vi "FGV Rel.vi"(5 "Extrem_Value":T1, 9 "action":enum16{"set", "get"}(ring), 11 "error in (no error)":errorcluster) -> (6 "Extrem_Value":T1, 15 "error out":errorcluster)   [LabVIEW 2014, in "FH 55.lvlib"]
uses:
  FH 55.lvlib
  TypeDef/Value_String.ctl
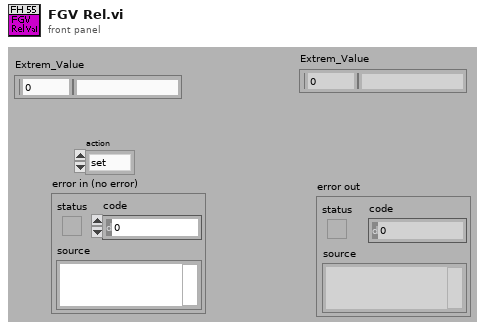
[diagram p1: front panel]
types:
  T1 = typedef "FH 55.lvlib/Value_String.ctl" = cluster{"Numeric":dbl, "String":string}
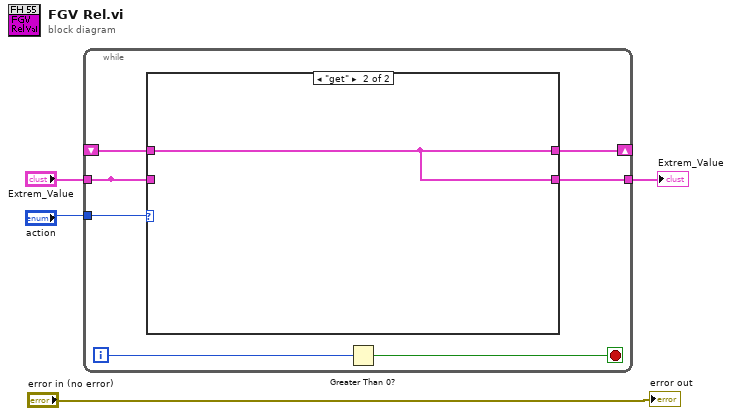
[diagram p0: block diagram]
diagram:
  n1 = while {
    tunnel: "Extrem_Value" -> [w10]
    tunnel: [w10] -> _
    shift-right: [w8] -> _
    shift-left: _ -> [w11]
    tunnel: [w9] -> w2
    tunnel: "action" -> [w5]
    i -> [w7]
    stop <- w6 stop-if-true
    n2 = case shown="\"get\"" w5 {
      tunnel: w11 -> [_ w13]
      tunnel: w10 -> [w12 _]
      tunnel: [w12 w13] -> w9
      tunnel: [w12 w13] -> w8
      frame "set", Default {
      }
      frame "get" {
      }
    }
    n3 = Greater Than 0?(x=w7) -> (x > 0?=w6:bool)
  }
  "Extrem_Value" <- w2
  "error out" <- "error in (no error)"
